vi "Update Monitor Label.vi"(8 "error in (no error)":errorcluster, 9 "Actor to Log":refnum<class "Message Enqueuer.lvclass">, 10 "Label":string, 11 "Classic Logger in":refnum<class "Classic Logger.lvclass">) -> (0 "error out":errorcluster, 3 "Classic Logger out":refnum<class "Classic Logger.lvclass">)   [LabVIEW 2023, in "Monitored Actor.lvlib" / "Classic Logger.lvclass"]
uses:
  Classic Logger.lvclass
  builds/Engine/Actor Framework.lvlibp/1abvi3w/vi.lib/ActorFramework/Message Enqueuer/Message Enqueuer.lvclass
  Classic Logger.lvclass/Classic Logger.ctl
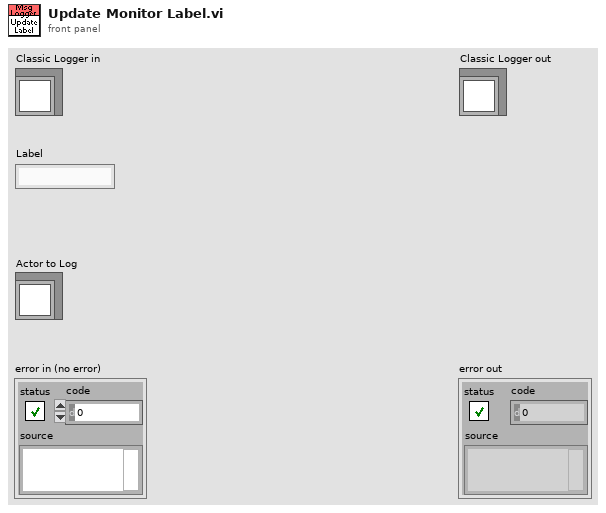
[diagram p1: front panel]
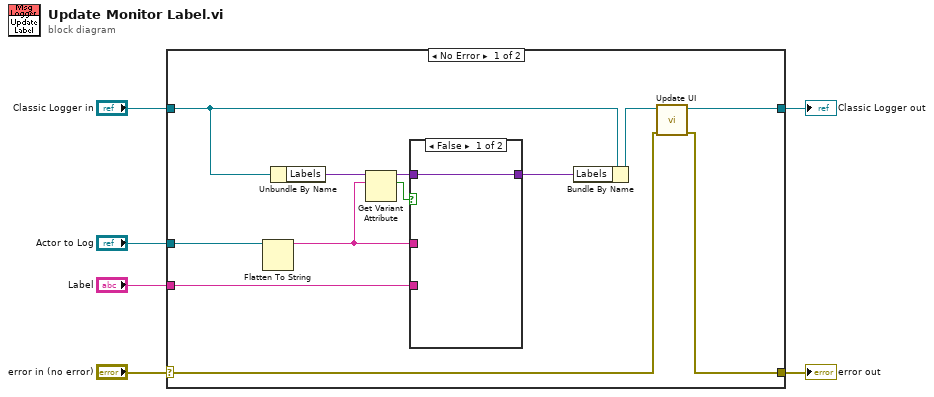
[diagram p0: block diagram]
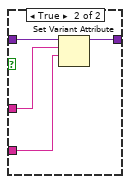
[diagram p2: hidden frame]
diagram:
  n1 = case shown="No Error" "error in (no error)" {
    selector: "error in (no error)" -> [w8 w25]
    tunnel: [w7 w25] -> w5
    tunnel: [w9 w24] -> w3
    tunnel: "Classic Logger in" -> [w18 w24]
    tunnel: "Actor to Log" -> [w16 _]
    tunnel: "Label" -> [w12 _]
    frame No Error {
      n2 = Flatten To String(anything=w16) -> (data string=w11:string)  [unwired: 3 in, 2 out]
      n3 = Unbundle By Name(w18) -> ("Labels"=w15:variant)
      n4 = Get Variant Attribute(Variant=w15, name=w11) -> (duplicate Variant=w14:variant, found=w10:bool)  [unwired: 2 in, 2 out]
      n5 = case shown="False" w10 {
        tunnel: w14 -> [w19 w23]
        tunnel: [w19 w22] -> w13
        tunnel: w12 -> [_ w21]
        tunnel: w11 -> [_ w20]
        frame False {
        }
        frame True {
          n6 = Set Variant Attribute(Variant=w23, name=w20, value=w21) -> (Variant out=w22:variant)  [unwired: 1 in, 2 out]
        }
      }
      n7 = Bundle By Name(cluster=w18, "Labels"=w13) -> (w17:refnum<class "Classic Logger.lvclass">)
      n8 = call "Update UI.vi"("error in (no error)"=w8, "Message Logger in"=w17) -> ("error out"=w7:errorcluster, "Message Logger out"=w9:refnum<class "Classic Logger.lvclass">)  [unwired: 8 in]
    }
    frame Error {
    }
  }
  "error out" <- w5
  "Classic Logger out" <- w3
